vi "ALONE_ALICATS.vi"(7 "Refresco(s)":dbl=5.0 caption="Elapsed Time (s)", 8 "error in (no error)":errorcluster) -> (0 "error out":errorcluster, 5 "Remote?":bool)   [LabVIEW 2017]
uses:
  SERIAL ALICATS/__s_TablaAlicats.ctl
  TIMING/Timing_Module Control.ctl
  SERIAL ALICATS/__Alicat SD_Hardware_Module.ctl
  REACTOR_GLOBALES.vi
panel:
  out "Numeric":dbl format="%.1f"
  out "ALICATS_NODES 2":T1
  out "Nodes":i32=5 caption="Elapsed Time (s)"
  out "ALICATS_UNITS":T2
  out "ALICATS_GASES":T2
  out "Delta (s)":dbl caption="Elapsed Time (s)" format="%.1f"
  out "CICLO":i32=5 caption="Elapsed Time (s)"
  in  "Write":bool
  out "Dispositivos":T3 caption="Alicat massflow"
  out "Date":string caption="asd"
  out "Time":string caption="asd"
  out "Tiempo (m)":dbl caption="Elapsed Time (s)" format="%.1f"
  in  "stop":bool
  out "Refresh":bool
  # "Control de flujos de gases"
  # "5"
  # "4"
  # "3"
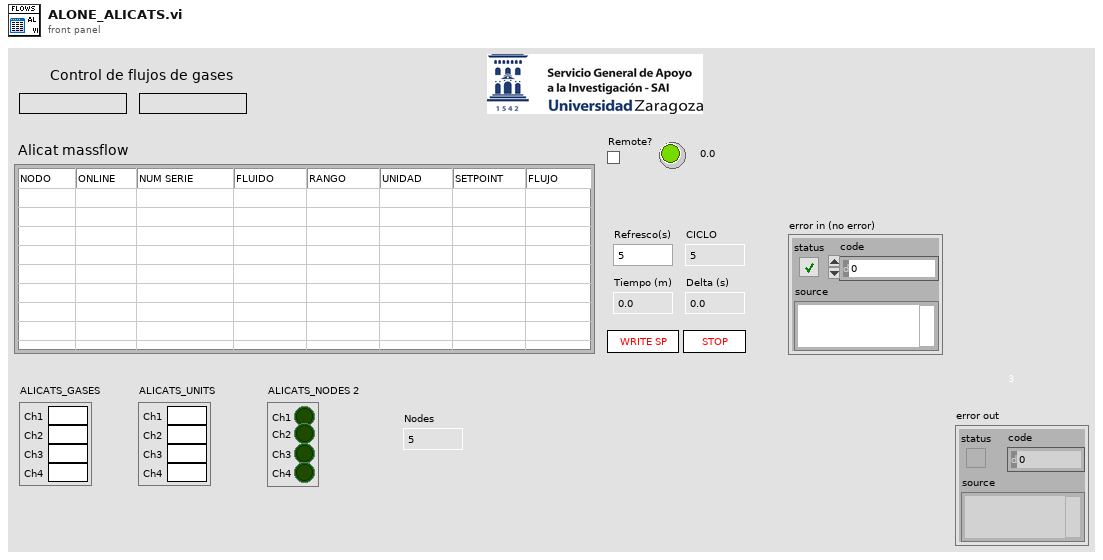
[diagram p1: front panel]
types:
  T1 = cluster{"Ch1":bool, "Ch2":bool, "Ch3":bool, "Ch4":bool}
  T2 = cluster{"Ch1":string, "Ch2":string, "Ch3":string, "Ch4":string}
  T3 = typedef "__s_TablaAlicats.ctl" = string[][]
  T4 = typedef "Timing_Module Control.ctl" = enum16{"Initialize Time", "Check Time"}
  T5 = typedef "__Alicat SD_Hardware_Module.ctl" = enum16{"Initialize", "Send Setpoint", "Read Data", "Change Address", "Shutdown"}
  T6 = typedef "REACTOR_COMUNICACIONES.ctl" = cluster{"Alicats":refnum<visa-resource-name>, "Alic":bool, "eValve":refnum<visa-resource-name>, "eval":bool, "Eurotherm":refnum<visa-resource-name>, "euro":bool, "Cell GAS":refnum<visa-resource-name>, "cgas":bool, "Cell H2S":refnum<visa-resource-name>, "ch2s":bool}
  T7 = typedef "__s_SPali4.ctl" = cluster{"Ch1":dbl, "Ch2":dbl, "Ch3":dbl, "Ch4":dbl}
  T8 = cluster{"[0]":bool, "[1]":bool, "[2]":bool, "[3]":bool}
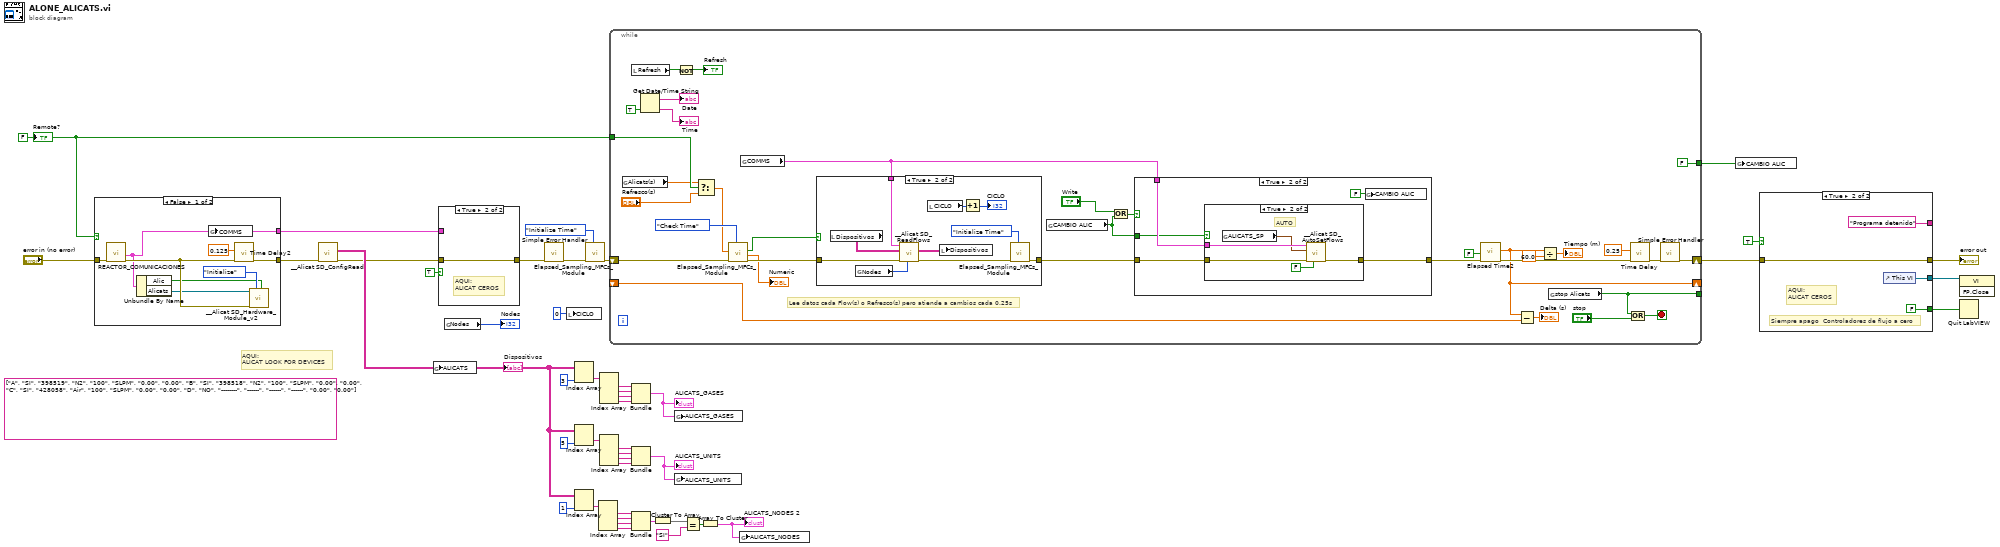
[diagram p0: block diagram]
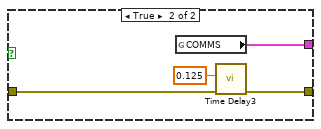
[diagram p2: hidden frame]
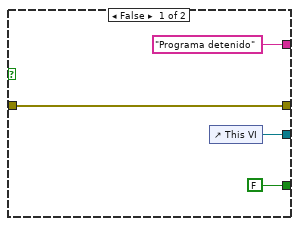
[diagram p4: hidden frame]
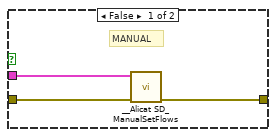
[diagram p7: hidden frame]
diagram:
  (unwired) T3 [["A", "SI", "398519", "N2", "100", "SLPM", "0.00", "0.00"], ["B", "SI", "398518", "N2", "100", "SLPM", "0.00", "0.00"], ["C", "SI", "428058", "Air", "100", "SLPM", "0.00", "0.00"], ["D", "NO", "--------", "------", "------", "------", "0.00", "0.00"]] ("aDispositivos")
  w38 = FALSE ("Remote?")
  # "AQUI:\nALICAT LOOK FOR DEVICES"
  n1 = case shown="False" w38 {
    tunnel: [w47 w53] -> w36
    tunnel: "error in (no error)" -> [w52 w55]
    tunnel: [w50 w54] -> w3
    frame False {
      n2 = call "REACTOR_COMUNICACIONES.vi"("error in (no error)"=w52) -> ("error out"=w48:errorcluster, "COMMS"=w47:T6)  [unwired: 8 in, 1 out]
      n3 = Unbundle By Name(w47) -> ("Alic"=w45:bool, "Alicats"=w46:refnum<visa-resource-name>)
      n4 = global write "REACTOR_GLOBALES.vi" "COMMS"(w47) -> ()
      n5 = call "Time Delay2"("error in (no error)"=w48, "Delay Time (s)"=0.125) -> ("error out"=w50:errorcluster)  [unwired: 9 in]
      n6 = call "__Alicat SD_Hardware_Module_v2.vi"("Used ?"=w45, "Command"=__Alicat_SD_Hardware_Module."Initialize", "error in (no error)"=w48, "VISA resource name"=w46) -> ()  [unwired: 4 in, 4 out]
    }
    frame True {
      n7 = global read "REACTOR_GLOBALES.vi" "COMMS"() -> (w53:T6)
      n8 = call "Time Delay3"("error in (no error)"=w55, "Delay Time (s)"=0.125) -> ("error out"=w54:errorcluster)  [unwired: 9 in]
    }
  }
  n9 = call "__Alicat SD_ConfigRead.vi"("error in (no error)"=w3) -> ("error out"=w2:errorcluster, "AlicatsControl"=w5:T3)  [unwired: 8 in]
  "Dispositivos" <- w5
  n10 = global write "REACTOR_GLOBALES.vi" "ALICATS"(w5) -> ()
  n11 = case shown="True" TRUE {
    tunnel: w2 -> [w57 w58]
    tunnel: [w57 w58] -> w19
    tunnel: w36 -> [_ _]
    frame False {
    }
    frame True {
      # "AQUI:\nALICAT CEROS"
    }
  }
  n12 = global read "REACTOR_GLOBALES.vi" "Nodes"() -> (→"Nodes":i32)
  n13 = call <vilib>:"Simple Error Handler.vi"("error in (no error)"=w19) -> ("error out"=w18:errorcluster)  [unwired: 4 in, 4 out]
  n14 = local write "CICLO"(0 ("CICLO")) -> ()
  n15 = Index Array(array=w5, index (col)=1 ("index")) -> (element=w15:string[])  [unwired: 1 in]
  n16 = Index Array(array=w5, index (col)=3 ("index")) -> (element=w34:string[])  [unwired: 1 in]
  n17 = Index Array(array=w5, index (col)=5 ("index")) -> (element=w25:string[])  [unwired: 1 in]
  n18 = call "Elapsed_Sampling_MFCs_Module.vi"("Command"=Timing_Module_Control."Initialize Time", "error in (no error)"=w18) -> ("error out"=w17:errorcluster)  [unwired: 7 in, 2 out]
  n19 = Index Array(array=w15) -> (element #1=w14:string, element #2=w13:string, element #3=w12:string, element #4=w11:string)  [unwired: 4 in]
  n20 = Index Array(array=w34) -> (element #1=w33:string, element #2=w32:string, element #3=w31:string, element #4=w30:string)  [unwired: 4 in]
  n21 = Index Array(array=w25) -> (element #1=w26:string, element #2=w27:string, element #3=w28:string, element #4=w29:string)  [unwired: 4 in]
  n22 = while {
    shift-right: [w85] -> w44
    shift-left: w17 -> [w68]
    tunnel: [w62] -> _
    tunnel: [FALSE ("stop")] -> w40
    tunnel: w38 -> [w79]
    shift-right: [w75] -> _
    shift-left: _ -> [w76]
    stop <- w92 stop-if-true
    # "Lee datos cada Flow(s) o Refresco(s) pero atiende a cambios cada 0.25s"
    n23 = global read "REACTOR_GLOBALES.vi" "Alicats(s)"() -> (w63:dbl)
    n24 = local read "Refresh"() -> (w86:bool)
    n25 = Get Date/Time String(want seconds? (F)=TRUE) -> (date string=→"Date":string, time string=→"Time":string)  [unwired: 2 in]
    n26 = Not(x=w86) -> (.not. x?=→"Refresh":bool)
    n27 = Select(t=w63, s=w79, f="Refresco(s)") -> (s? t:f=w69:dbl)
    n28 = call "Elapsed_Sampling_MFCs_Module.vi"("Command"=Timing_Module_Control."Check Time", "error in (no error)"=w68, "Time In"=w69) -> ("error out"=w67:errorcluster, "Elapsed Out"=→"Numeric":dbl, "Time Elapsed"=w66:bool)  [unwired: 6 in]
    n29 = global read "REACTOR_GLOBALES.vi" "COMMS"() -> (w61:T6)
    n30 = case shown="True" w66 {
      tunnel: w61 -> [_ w97]
      tunnel: [w93 w102] -> w64
      tunnel: w67 -> [w93 w101]
      frame False {
      }
      frame True {
        n31 = local read "Dispositivos"() -> (w96:T3)
        n32 = global read "REACTOR_GLOBALES.vi" "Nodes"() -> (w98:i32)
        n33 = call "__Alicat SD_ReadFlows.vi"("Nodos"=w98, "error in"=w101, "aDispositivos"=w96, "COMMS"=w97) -> ("error out"=w99:errorcluster, "aDispositivos 2"=w100:T3)  [unwired: 5 in, 1 out]
        n34 = local read "CICLO"() -> (w94:i32)
        n35 = local write "Dispositivos"(w100) -> ()
        n36 = Increment(x=w94) -> (x+1=→"CICLO":i32)
        n37 = call "Elapsed_Sampling_MFCs_Module.vi"("Command"=Timing_Module_Control."Initialize Time", "error in (no error)"=w99) -> ("error out"=w102:errorcluster)  [unwired: 7 in, 2 out]
      }
    }
    n38 = global read "REACTOR_GLOBALES.vi" "CAMBIO ALIC"() -> (w60:bool)
    n39 = Or(x="Write", y=w60) -> (x .or. y?=w71:bool)
    n40 = case shown="True" w71 {
      tunnel: [w104 w107] -> w73
      tunnel: w64 -> [w104 w108]
      tunnel: w61 -> [_ w106]
      tunnel: w60 -> [_ w105]
      frame False {
      }
      frame True {
        n41 = case shown="True" w105 {
          tunnel: w108 -> [w112 w117]
          tunnel: [w111 w116] -> w107
          tunnel: w106 -> [w110 w115]
          frame False {
            # "MANUAL"
            n42 = call "__Alicat SD_ManualSetFlows.vi"("error in (no error)"=w112, "COMMS"=w110) -> ("error out"=w111:errorcluster)  [unwired: 6 in, 1 out]
          }
          frame True {
            # "AUTO"
            n43 = global read "REACTOR_GLOBALES.vi" "ALICATS_SP"() -> (w114:T7)
            n44 = call "__Alicat SD_AutoSetFlows.vi"("Cero"=FALSE, "error in (no error)"=w117, "ALICATS_SP"=w114, "COMMS"=w115) -> ("error out"=w116:errorcluster)  [unwired: 7 in]
          }
        }
        n45 = global write "REACTOR_GLOBALES.vi" "CAMBIO ALIC"(FALSE ("ChangeF")) -> ()
      }
    }
    n46 = call "Elapsed Time2"("Auto Reset"=FALSE, "error in (no error)"=w73) -> ("Elapsed Time (s)"=w75:dbl, "error out"=w84:errorcluster)  [unwired: 10 in, 6 out]
    n47 = Subtract(x=w75, y=w76) -> (x-y=→"Delta (s)":dbl)
    n48 = Divide(x=w75, y=60.0) -> (x/y=→"Tiempo (m)":dbl)
    n49 = global read "REACTOR_GLOBALES.vi" "stop Alicats"() -> (w62:bool)
    n50 = Or(x=w62, y="stop") -> (x .or. y?=w92:bool)
    n51 = call "Time Delay"("error in (no error)"=w84, "Delay Time (s)"=0.25) -> ("error out"=w83:errorcluster)  [unwired: 9 in]
    n52 = call <vilib>:"Simple Error Handler.vi"("error in (no error)"=w83) -> ("error out"=w85:errorcluster)  [unwired: 4 in, 4 out]
  }
  n53 = Bundle(w14, w13, w12, w11) -> (w7:cluster{string, string, string, string})  [unwired: 1 in]
  n54 = Bundle(w33, w32, w31, w30) -> (w22:cluster{string, string, string, string})  [unwired: 1 in]
  "ALICATS_GASES" <- w22
  n55 = Bundle(w26, w27, w28, w29) -> (w23:cluster{string, string, string, string})  [unwired: 1 in]
  "ALICATS_UNITS" <- w23
  n56 = Cluster To Array(cluster=w7) -> (array=w9:string[])
  n57 = global write "REACTOR_GLOBALES.vi" "ALICATS_GASES"(w22) -> ()
  n58 = global write "REACTOR_GLOBALES.vi" "ALICATS_UNITS"(w23) -> ()
  n59 = Equal?(x=w9, y="SI") -> (x = y?=w10:bool[])
  n60 = Array To Cluster(array=w10) -> (cluster=w6:T8)
  "ALICATS_NODES 2" <- w6
  n61 = global write "REACTOR_GLOBALES.vi" "ALICATS_NODES"(w6) -> ()
  n62 = global write "REACTOR_GLOBALES.vi" "CAMBIO ALIC"(w40) -> ()
  n63 = case shown="True" TRUE {
    tunnel: w44 -> [w120 w122]
    tunnel: [w120 w122] -> w43
    tunnel: ["Programa detenido" ("message") "Programa detenido" ("message")] -> _
    tunnel: [FALSE FALSE] -> w41
    tunnel: [w118 w123] -> w39
    frame False {
      n64 = control-ref of="This VI"() -> (w118:refnum<vi>)
    }
    frame True {
      # "AQUI:\nALICAT CEROS"
      # "Siempre apago  Controladores de flujo a cero"
      n65 = control-ref of="This VI"() -> (w123:refnum<vi>)
    }
  }
  "error out" <- w43
  n66 = invoke class="VI" method="FP.Close"(reference=w39) -> ()  [unwired: 2 in, 3 out]
  n67 = Quit LabVIEW(quit? (T)=w41) -> ()
  "Remote?" <- w38
